vi "GenerateLine.vi"(1 "Color":u32(colorbox)=13421772, 2 "Frame End":T1={"nx"=1.0, "ny"=0.0, "nz"=0.0, "nw"=0.0, "ox"=0.0, "oy"=1.0, "oz"=0.0, "ow"=0.0, "ax"=0.0, "ay"=0.0, "az"=1.0, "aw"=0.0, "Px"=0.0, "Py"=0.0, "Pz"=0.0, "Pw"=1.0} {"Pw" format="%.2f"; "Pz" format="%.2f"; "Py" format="%.2f"; "Px" format="%.2f"; "aw" format="%.2f"; "az" format="%.2f"; "ay" format="%.2f"; "ax" format="%.2f"; "ow" format="%.2f"; "nw" format="%.2f"; "oz" format="%.2f"; "oy" format="%.2f"; "ox" format="%.2f"; "nz" format="%.2f"; "ny" format="%.2f"; "nx" format="%.2f"}, 3 "Frame Start":T1={"nx"=1.0, "ny"=0.0, "nz"=0.0, "nw"=0.0, "ox"=0.0, "oy"=1.0, "oz"=0.0, "ow"=0.0, "ax"=0.0, "ay"=0.0, "az"=1.0, "aw"=0.0, "Px"=0.0, "Py"=0.0, "Pz"=0.0, "Pw"=1.0} {"Pw" format="%.2f"; "Pz" format="%.2f"; "Py" format="%.2f"; "Px" format="%.2f"; "aw" format="%.2f"; "az" format="%.2f"; "ay" format="%.2f"; "ax" format="%.2f"; "ow" format="%.2f"; "nw" format="%.2f"; "oz" format="%.2f"; "oy" format="%.2f"; "ox" format="%.2f"; "nz" format="%.2f"; "ny" format="%.2f"; "nx" format="%.2f"}, 4 "Text In":string) -> (0 "Text Out":string="Shape {\nappearance Appearance {\nmaterial Material {\nemissiveColor 0.80 0.80 0.80\n}\n}\ngeometry IndexedLineSet {\ncoord Coordinate {\npoint [\n0.00 0.00 0.00,0.00 0.00 0.00]}\ncoordIndex [0, 1\r]}}")   [LabVIEW 2012]
uses:
  <userlib>/rosforlv/Gazebo/AxesDrawing/ReferenceFrame.ctl
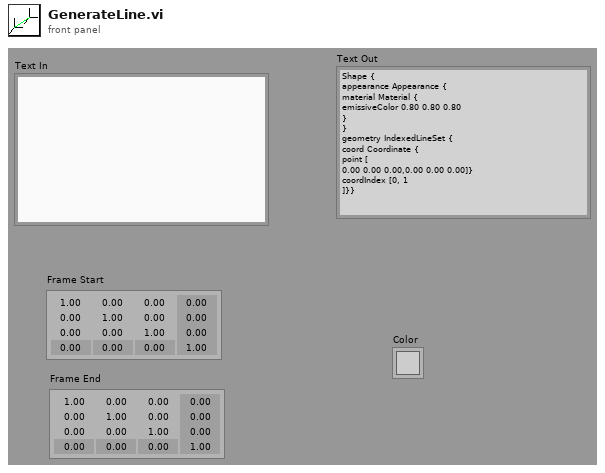
[diagram p1: front panel]
types:
  T1 = typedef "ReferenceFrame.ctl" = cluster{"nx":dbl, "ny":dbl, "nz":dbl, "nw":dbl, "ox":dbl, "oy":dbl, "oz":dbl, "ow":dbl, "ax":dbl, "ay":dbl, "az":dbl, "aw":dbl, "Px":dbl, "Py":dbl, "Pz":dbl, "Pw":dbl}
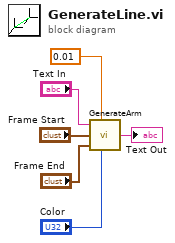
[diagram p0: block diagram]
diagram:
  n1 = call <userlib>:"GenerateArm.vi"("Text In"="Text In", "Arm Width"=0.01, "Frame Start"="Frame Start", "Frame End"="Frame End", "Color"="Color") -> ("Text Out"=→"Text Out":string)
